vi "Build string table (excel).vi"(1 "row headers":string[](array[string]), 2 "column headers":string[](array[string]), 3 "text data":string[][](array[string])) -> (0 "output table":string[][](array[string]))   [LabVIEW 2010, in "NI_ReportGenerationToolkit.lvlib"]
uses:
  <vilib>/addons/_office/NI_ReportGenerationToolkit.lvlib
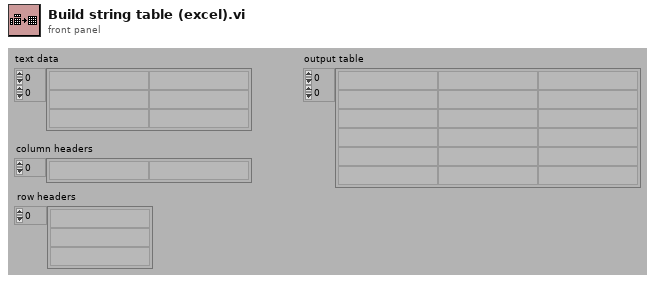
[diagram p1: front panel]
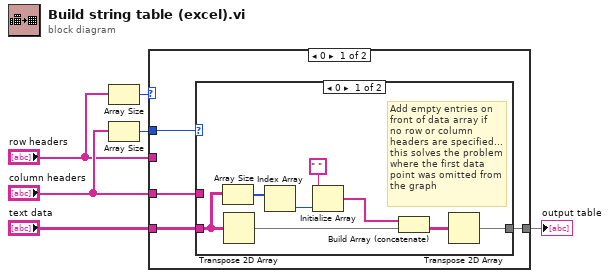
[diagram p0: block diagram]
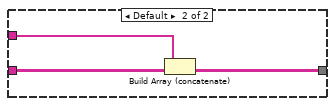
[diagram p2: hidden frame]
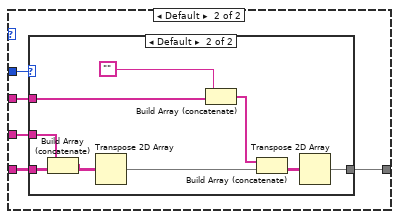
[diagram p3: hidden frame]
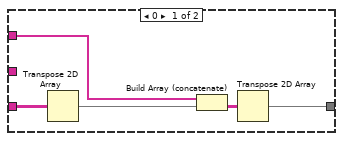
[diagram p4: hidden frame]
diagram:
  n1 = Array Size(array="row headers") -> (size(s)=w2:i32)
  n2 = Array Size(array="column headers") -> (size(s)=w1:i32)
  n3 = case shown="0" w2 {
    tunnel: [w7 w26] -> w6
    tunnel: "column headers" -> [w9 w25]
    tunnel: w1 -> [w10 w24]
    tunnel: "text data" -> [w8 w23]
    tunnel: "row headers" -> [_ w22]
    frame 0 {
      n4 = case shown="0" w10 {
        tunnel: w9 -> [_ w21]
        tunnel: w8 -> [w15 w20]
        tunnel: [w16 w19] -> w7
        frame 0 {
          # "Add empty entries on\nfront of data array if\nno row or column \nheaders are specified...\nthis solves the problem\nwhere the first data \npoint was omitted from\nthe graph"
          n5 = Array Size(array=w15) -> (size(s)=w14:i32[])
          n6 = Transpose 2D Array(2D array=w15) -> (transposed array=w17:string[][])
          n7 = Index Array(array=w14) -> (element=w13:i32)  [unwired: 1 in]
          n8 = Initialize Array(" ", w13) -> (w12:string[])
          n9 = Build Array (concatenate)(w12, w17) -> (w18:string[][])
          n10 = Transpose 2D Array(2D array=w18) -> (transposed array=w16:string[][])
        }
        frame Default {
          n11 = Build Array (concatenate)(w21, w20) -> (w19:string[][])
        }
      }
    }
    frame Default {
      n12 = case shown="Default" w24 {
        tunnel: [w28 w38] -> w26
        tunnel: w25 -> [_ w35]
        tunnel: w23 -> [w30 w34]
        tunnel: w22 -> [w31 w32]
        frame 0 {
          n13 = Transpose 2D Array(2D array=w30) -> (transposed array=w29:string[][])
          n14 = Build Array (concatenate)(w31, w29) -> (w27:string[][])
          n15 = Transpose 2D Array(2D array=w27) -> (transposed array=w28:string[][])
        }
        frame Default {
          n16 = Build Array (concatenate)(w35, w34) -> (w33:string[][])
          n17 = Transpose 2D Array(2D array=w33) -> (transposed array=w37:string[][])
          n18 = Build Array (concatenate)("", w32) -> (w36:string[])
          n19 = Build Array (concatenate)(w36, w37) -> (w39:string[][])
          n20 = Transpose 2D Array(2D array=w39) -> (transposed array=w38:string[][])
        }
      }
    }
  }
  "output table" <- w6
